vi "AD Open Motors (Drivebase).vi"(1 "PID Constants for Sparks":T1={"P Gain"=0.00035, "I Gain"=5e-07, "D Gain"=0.0, "F Gain"=0.0002, "I Zone"=0.0, "Min Output"=-1.0, "Max Output"=1.0}) -> (0 "output cluster":cluster{"Left":string[], "Right":string[]})   [LabVIEW 2019]
uses:
  <vilib>/Rock Robotics/WPI/ThirdParty/REV Robotics/SPARK MAX/Typedef/Spark MAX Idle Mode.ctl
  2020 Robot/Framework/Robot Global Data.vi
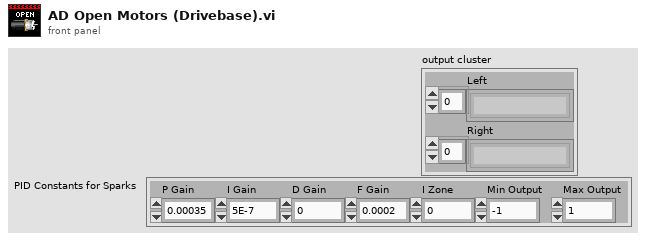
[diagram p1: front panel]
types:
  T1 = cluster{"P Gain":dbl, "I Gain":dbl, "D Gain":dbl, "F Gain":dbl, "I Zone":dbl, "Min Output":dbl, "Max Output":dbl}
  T2 = typedef "Spark MAX Idle Mode.ctl" = enum16{"Coast", "Brake"}
  T3 = typedef "WPI_MotorControlDeviceRef.ctl" = cluster{"DeviceStatus":errorcluster, "Type":T4, "PWM":cluster{"PWM Channel":T5, "DeadBand":T6}, "CAN":cluster{"Device Number":u8, "SetOutput VI Ref":variant, "GetOutput VI Ref":variant, "Enable VI Ref":variant, "Disable VI Ref":variant, "Data":variant}, "Invert":bool, "DIO PWM":cluster{"PWM \"Enable\" Channel":T5, "DIOChannel":T7, "PWM Rate":dbl}}
  T4 = typedef "WPI_MotorControlType.ctl" = enum16{"PWM", "CAN", "DIO PWM"}
  T5 = typedef "FPGA_DIOPWMChannel.ctl" = enum8{"PWM 0", "PWM 1", "PWM 2", "PWM 3", "PWM 4", "PWM 5", "PWM 6", "PWM 7", "PWM 8", "PWM 9", "PWM MXP 0", "PWM MXP 1", "PWM MXP 2", "PWM MXP 3", "PWM MXP 4", "PWM MXP 5", "PWM MXP 6", "PWM MXP 7", "PWM MXP 8", "PWM MXP 9", "Invalid"}
  T6 = typedef "WPI_PWMDeadband.ctl" = cluster{"Name":string, "maxPositivePwm":i32, "minPositivePwm":i32, "centerPwm":i32, "maxNegativePwm":i32, "minNegativePwm":i32, "angularRange":u16}
  T7 = typedef "FPGA_DIOChannel.ctl" = enum8{"DIO 0", "DIO 1", "DIO 2", "DIO 3", "DIO 4", "DIO 5", "DIO 6", "DIO 7", "DIO 8", "DIO 9", "DIO MXP 0", "DIO MXP 1", "DIO MXP 2", "DIO MXP 3", "DIO MXP 4", "DIO MXP 5", "DIO MXP 6", "DIO MXP 7", "DIO MXP 8", "DIO MXP 9", "DIO MXP 10", "DIO MXP 11", "DIO MXP 12", "DIO MXP 13", "DIO MXP 14", "DIO MXP 15", "SPI Port CS1", "SPI Port CS2", "SPI Port CS3", "SPI Port MISO", "SPI Port MOSI", "Invalid"}
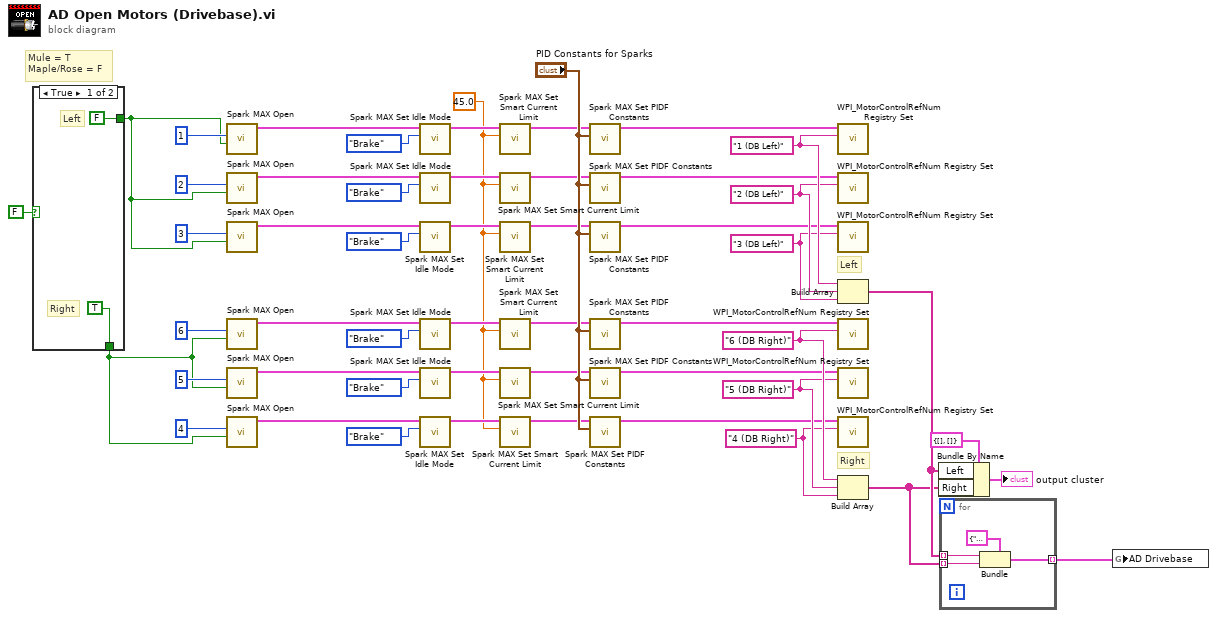
[diagram p0: block diagram]
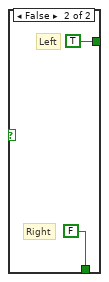
[diagram p2: hidden frame]
diagram:
  w4 = sgl 45.0 ("Current Limit A (100)")
  w41 = "4 (DB Right)" ("refnum name")
  w42 = "5 (DB Right)" ("refnum name")
  w43 = "6 (DB Right)" ("refnum name")
  w44 = "3 (DB Left)" ("refnum name")
  w45 = "2 (DB Left)" ("refnum name")
  w46 = "1 (DB Left)" ("refnum name")
  # "Mule = T\nMaple/Rose = F"
  # "Left"
  # "Right"
  n1 = case shown="True" FALSE {
    tunnel: [FALSE ("Invert") TRUE ("Invert")] -> w3
    tunnel: [TRUE ("Invert") FALSE ("Invert")] -> w2
    frame True {
      # "Right"
      # "Left"
    }
    frame False {
      # "Right"
      # "Left"
    }
  }
  n2 = call <vilib>:"Spark MAX Open.vi"("Invert"=w3, "Device Number"=u8 1) -> ("MotorControlDeviceRef"=w32:T3)  [unwired: 8 in, 1 out]
  n3 = call <vilib>:"Spark MAX Open.vi"("Invert"=w3, "Device Number"=u8 2) -> ("MotorControlDeviceRef"=w31:T3)  [unwired: 8 in, 1 out]
  n4 = call <vilib>:"Spark MAX Open.vi"("Invert"=w3, "Device Number"=u8 3) -> ("MotorControlDeviceRef"=w30:T3)  [unwired: 8 in, 1 out]
  n5 = call <vilib>:"Spark MAX Open.vi"("Invert"=w2, "Device Number"=u8 6) -> ("MotorControlDeviceRef"=w29:T3)  [unwired: 8 in, 1 out]
  n6 = call <vilib>:"Spark MAX Open.vi"("Invert"=w2, "Device Number"=u8 5) -> ("MotorControlDeviceRef"=w28:T3)  [unwired: 8 in, 1 out]
  n7 = call <vilib>:"Spark MAX Open.vi"("Invert"=w2, "Device Number"=u8 4) -> ("MotorControlDeviceRef"=w27:T3)  [unwired: 8 in, 1 out]
  n8 = call <vilib>:"Spark MAX Set Idle Mode.vi"("Idle Mode"=Spark_MAX_Idle_Mode."Brake", "MotorControlDeviceRef in"=w32) -> ("MotorControlDeviceRef out"=w16:T3)  [unwired: 8 in, 1 out]
  n9 = call <vilib>:"Spark MAX Set Idle Mode.vi"("Idle Mode"=Spark_MAX_Idle_Mode."Brake", "MotorControlDeviceRef in"=w31) -> ("MotorControlDeviceRef out"=w15:T3)  [unwired: 8 in, 1 out]
  n10 = call <vilib>:"Spark MAX Set Idle Mode.vi"("Idle Mode"=Spark_MAX_Idle_Mode."Brake", "MotorControlDeviceRef in"=w30) -> ("MotorControlDeviceRef out"=w14:T3)  [unwired: 8 in, 1 out]
  n11 = call <vilib>:"Spark MAX Set Idle Mode.vi"("Idle Mode"=Spark_MAX_Idle_Mode."Brake", "MotorControlDeviceRef in"=w29) -> ("MotorControlDeviceRef out"=w13:T3)  [unwired: 8 in, 1 out]
  n12 = call <vilib>:"Spark MAX Set Idle Mode.vi"("Idle Mode"=Spark_MAX_Idle_Mode."Brake", "MotorControlDeviceRef in"=w28) -> ("MotorControlDeviceRef out"=w12:T3)  [unwired: 8 in, 1 out]
  n13 = call <vilib>:"Spark MAX Set Idle Mode.vi"("Idle Mode"=Spark_MAX_Idle_Mode."Brake", "MotorControlDeviceRef in"=w27) -> ("MotorControlDeviceRef out"=w11:T3)  [unwired: 8 in, 1 out]
  n14 = call <vilib>:"Spark MAX Set Smart Current Limit.vi"("Primay Current Limit (80A)"=w4, "MotorControlDeviceRef in"=w16) -> ("MotorControlDeviceRef out"=w10:T3)  [unwired: 8 in, 1 out]
  n15 = call <vilib>:"Spark MAX Set Smart Current Limit.vi"("Primay Current Limit (80A)"=w4, "MotorControlDeviceRef in"=w15) -> ("MotorControlDeviceRef out"=w9:T3)  [unwired: 8 in, 1 out]
  n16 = call <vilib>:"Spark MAX Set Smart Current Limit.vi"("Primay Current Limit (80A)"=w4, "MotorControlDeviceRef in"=w14) -> ("MotorControlDeviceRef out"=w8:T3)  [unwired: 8 in, 1 out]
  n17 = call <vilib>:"Spark MAX Set Smart Current Limit.vi"("Primay Current Limit (80A)"=w4, "MotorControlDeviceRef in"=w13) -> ("MotorControlDeviceRef out"=w7:T3)  [unwired: 8 in, 1 out]
  n18 = call <vilib>:"Spark MAX Set Smart Current Limit.vi"("Primay Current Limit (80A)"=w4, "MotorControlDeviceRef in"=w12) -> ("MotorControlDeviceRef out"=w6:T3)  [unwired: 8 in, 1 out]
  n19 = call <vilib>:"Spark MAX Set Smart Current Limit.vi"("Primay Current Limit (80A)"=w4, "MotorControlDeviceRef in"=w11) -> ("MotorControlDeviceRef out"=w5:T3)  [unwired: 8 in, 1 out]
  n20 = call <vilib>:"Spark MAX Set PIDF Constants.vi"("PID Constants"="PID Constants for Sparks", "MotorControlDeviceRef"=w10) -> ("MotorControlDeviceRef"=w23:T3)  [unwired: 8 in, 1 out]
  n21 = call <vilib>:"Spark MAX Set PIDF Constants.vi"("PID Constants"="PID Constants for Sparks", "MotorControlDeviceRef"=w9) -> ("MotorControlDeviceRef"=w22:T3)  [unwired: 8 in, 1 out]
  n22 = call <vilib>:"Spark MAX Set PIDF Constants.vi"("PID Constants"="PID Constants for Sparks", "MotorControlDeviceRef"=w8) -> ("MotorControlDeviceRef"=w21:T3)  [unwired: 8 in, 1 out]
  n23 = call <vilib>:"Spark MAX Set PIDF Constants.vi"("PID Constants"="PID Constants for Sparks", "MotorControlDeviceRef"=w7) -> ("MotorControlDeviceRef"=w20:T3)  [unwired: 8 in, 1 out]
  n24 = call <vilib>:"Spark MAX Set PIDF Constants.vi"("PID Constants"="PID Constants for Sparks", "MotorControlDeviceRef"=w6) -> ("MotorControlDeviceRef"=w19:T3)  [unwired: 8 in, 1 out]
  n25 = call <vilib>:"Spark MAX Set PIDF Constants.vi"("PID Constants"="PID Constants for Sparks", "MotorControlDeviceRef"=w5) -> ("MotorControlDeviceRef"=w18:T3)  [unwired: 8 in, 1 out]
  n26 = call <vilib>:"WPI_MotorControlRefNum Registry Set.vi"("refnum name"=w46, "MotorControlDevRef"=w23) -> ()  [unwired: 8 in, 2 out]
  n27 = call <vilib>:"WPI_MotorControlRefNum Registry Set.vi"("refnum name"=w45, "MotorControlDevRef"=w22) -> ()  [unwired: 8 in, 2 out]
  n28 = call <vilib>:"WPI_MotorControlRefNum Registry Set.vi"("refnum name"=w44, "MotorControlDevRef"=w21) -> ()  [unwired: 8 in, 2 out]
  n29 = Build Array(w46, w45, w44) -> (w26:string[])
  n30 = call <vilib>:"WPI_MotorControlRefNum Registry Set.vi"("refnum name"=w43, "MotorControlDevRef"=w20) -> ()  [unwired: 8 in, 2 out]
  n31 = call <vilib>:"WPI_MotorControlRefNum Registry Set.vi"("refnum name"=w42, "MotorControlDevRef"=w19) -> ()  [unwired: 8 in, 2 out]
  n32 = call <vilib>:"WPI_MotorControlRefNum Registry Set.vi"("refnum name"=w41, "MotorControlDevRef"=w18) -> ()  [unwired: 8 in, 2 out]
  n33 = Build Array(w43, w42, w41) -> (w25:string[])
  n34 = Bundle By Name(cluster=cluster{"Left":string[], "Right":string[]} {"Left"=[], "Right"=[]} ("input cluster"), "Left"=w26, "Right"=w25) -> (→"output cluster":cluster{"Left":string[], "Right":string[]})
  n35 = for {
    tunnel: w26 -> [w60] mode=indexing
    tunnel: w25 -> [w59] mode=indexing
    tunnel: [w58] -> w24 mode=indexing
    n36 = Bundle(cluster=cluster{"Left":string, "Right":string} {"Left"="", "Right"=""} ("AD Drivebase"), "Left"=w60, "Right"=w59) -> (w58:cluster{"Left":string, "Right":string})
  }
  n37 = global write "Robot Global Data.vi" "AD Drivebase"(w24) -> ()
